vi "ConfigPhases.vi"(8 "error in (no error)":errorcluster, 11 "NhRegenGridSim in":refnum<class "NhRegenGridSim.lvclass">) -> (0 "error out":errorcluster, 3 "NhRegenGridSim out":refnum<class "NhRegenGridSim.lvclass">)   [LabVIEW 2018, in "AcPwrPlugins.lvlib" / "NhRegenGridSim.lvclass"]
doc: "This VI sets the selected logical instrument to apply changes at the set phase angle when operating with synchronization enabled using Configure Synchronization.vi.\n\nThis command ONLY applies to an instrument in AC mode."
uses:
  NhRegenGridSim.lvclass
  <instrlib>/NH Research 9400 Series/NH Research 9400 Series.lvlib
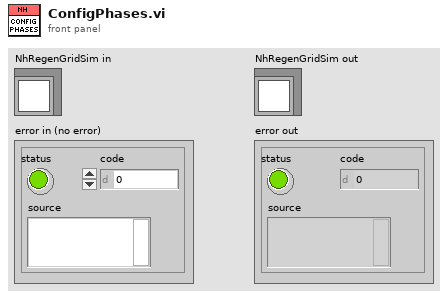
[diagram p1: front panel]
types:
  T1 = typedef "AcPwrPlugins.lvlib/NhRegenGridSim.lvclass/Load.ctl" = cluster{"SlewRates":cluster{"Islew":dbl, "Vslew":dbl, "Pslew":dbl, "FreqSlew":dbl, "AngleABSlew":dbl, "AngleACSlew":dbl}, "Phases":cluster{"Pout":dbl, "Iout":dbl, "PhaseAngle":dbl, "Vout":dbl, "Phase Name":string}[], "Measurement":cluster{"ApertureLength":dbl, "NumberOfSamples":u32}, "Ranges":cluster{"Irange":dbl, "Vrange":dbl}, "Mode":enum8{"One 3-Phase AC", "One AC", "One DC", "Three AC", "Three DC", "One 2-Phase AC and One AC", "One 2-Phase AC and One DC", "Two AC", "One AC and One DC", "Two AC and One DC", "One AC and Two DC", "One DC and One AC", "Two DC"}, "PowerMax":u16, "TransformerRatio":dbl, "Waveshape":dbl[], "Handle":string, "FreqOut":dbl, "Connected":bool, "Safety Limits":cluster{"Minimum Voltage (V)":dbl, "Minimum Voltage Time (s)":dbl, "Maximum Voltage (V)":dbl, "Maximum Voltage Time (s)":dbl, "Maximum Source Amps (A)":dbl, "Maximum Source Amps Time (s)":dbl, "Maximum Sink Amps (A)":dbl, "Maximum Sink Amps Time (s)":dbl, "Maximum Source Power (W)":dbl, "Maximum Source Power Time (s)":dbl, "Maximum Sink Power (W)":dbl, "Maximum Sink Power Time (s)":dbl, "Peak Voltage (V)":dbl, "Peak Voltage Enable":bool, "Peak Amps (A)":dbl, "Peak Amps Enable":bool}}
  T2 = enum8{"One 3-Phase AC", "One AC", "One DC", "Three AC", "Three DC", "One 2-Phase AC and One AC", "One 2-Phase AC and One DC", "Two AC", "One AC and One DC", "Two AC and One DC", "One AC and Two DC", "One DC and One AC", "Two DC"}
  T3 = cluster{"Pout":dbl, "Iout":dbl, "PhaseAngle":dbl, "Vout":dbl, "Phase Name":string}[]
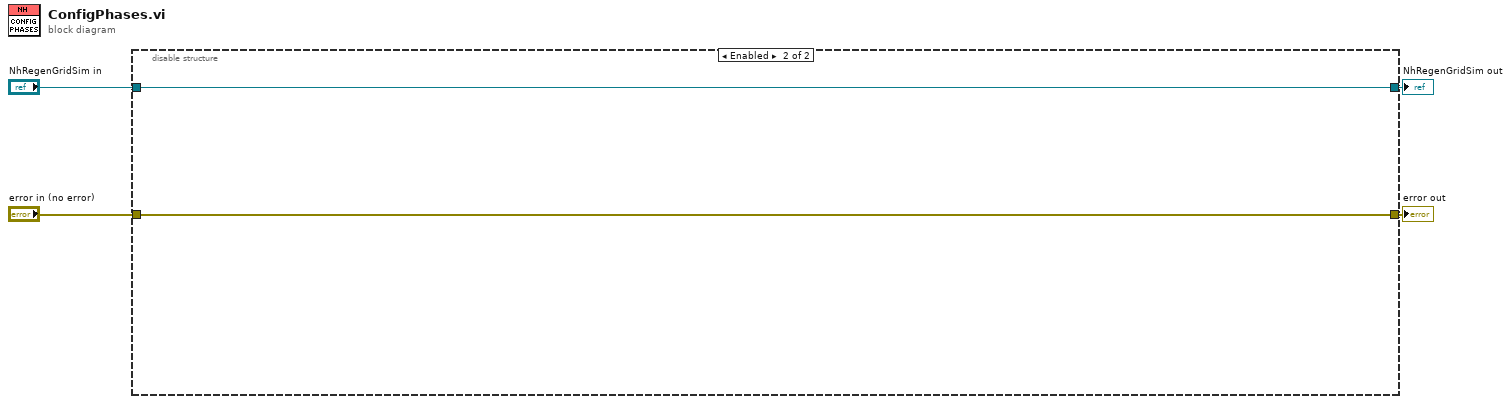
[diagram p0: block diagram]
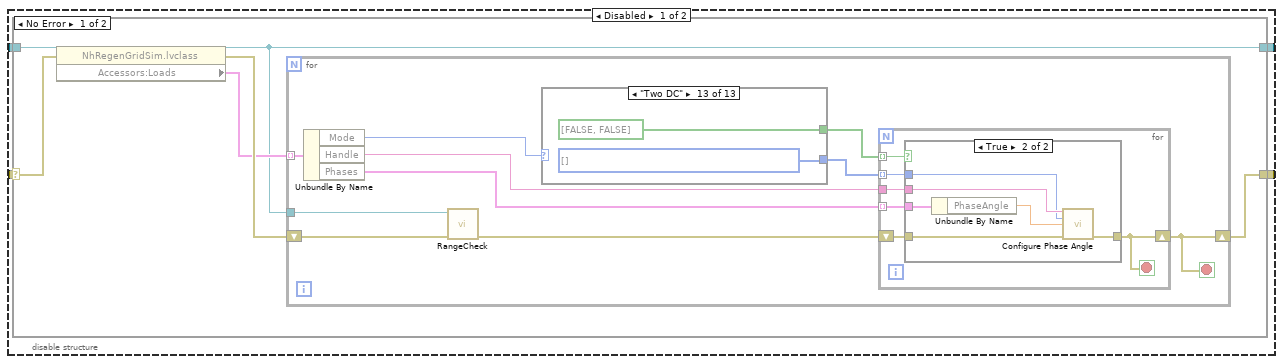
[diagram p2: hidden frame]
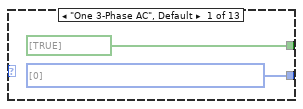
[diagram p3: hidden frame]
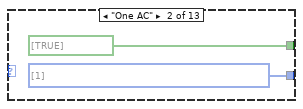
[diagram p4: hidden frame]
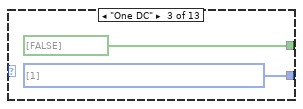
[diagram p5: hidden frame]
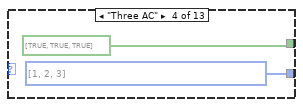
[diagram p6: hidden frame]
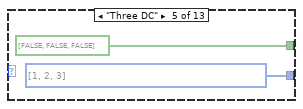
[diagram p7: hidden frame]
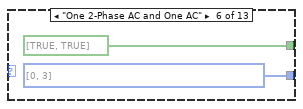
[diagram p8: hidden frame]
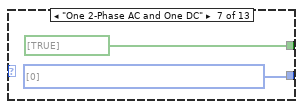
[diagram p9: hidden frame]
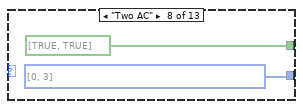
[diagram p10: hidden frame]
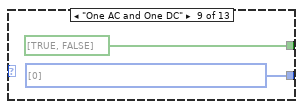
[diagram p11: hidden frame]
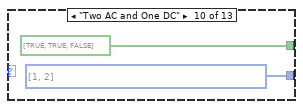
[diagram p12: hidden frame]
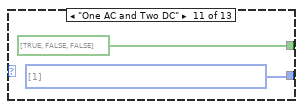
[diagram p13: hidden frame]
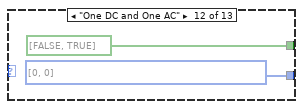
[diagram p14: hidden frame]
diagram:
  n1 = disable-structure shown="Enabled" {
    disable-tunnel: [w8 w66] -> w4
    disable-tunnel: [w7 w67] -> w3
    disable-tunnel: "error in (no error)" -> [w6 w66]
    disable-tunnel: "NhRegenGridSim in" -> [w5 w67]
    frame Disabled {
      n2 = case shown="No Error" w6 {
        selector: w6 -> [w13 w64]
        tunnel: [w11 w64] -> w8
        tunnel: [w9 w65] -> w7
        tunnel: w5 -> [w14 w65]
        frame No Error {
          n3 = property class="NhRegenGridSim.lvclass"(reference=w14, error in=w13) -> (reference out=w9:refnum<class "NhRegenGridSim.lvclass">, error out=w12:errorcluster, "Accessors:Loads"=w10:T1[])
          n4 = for {
            shift-right: [w18] -> w11
            shift-left: w12 -> [w21]
            tunnel: w10 -> [w23] mode=indexing
            tunnel: w9 -> [w19]
            stop <- w18 stop-if-true
            n5 = Unbundle By Name(w23) -> ("Mode"=w17:T2, "Handle"=w22:string, "Phases"=w24:T3)
            n6 = call-dynamic "RangeCheck.vi"("NhRegenGridSim in"=w19, "error in (no error)"=w21) -> ("error out"=w20:errorcluster)  [unwired: 7 in, 1 out]
            n7 = case shown="\"Two DC\"" w17 {
              tunnel: [w25 w28 w29 w32 w33 w35 w37 w39 w41 w43 w46 w48 w49] -> w15
              tunnel: [bool[] [TRUE] bool[] [TRUE] bool[] [FALSE] bool[] [TRUE, TRUE, TRUE] bool[] [FALSE, FALSE, FALSE] bool[] [TRUE, TRUE] bool[] [TRUE] bool[] [TRUE, TRUE] bool[] [TRUE, FALSE] bool[] [TRUE, TRUE, FALSE] bool[] [TRUE, FALSE, FALSE] bool[] [FALSE, TRUE] bool[] [FALSE, FALSE]] -> w16
              frame "One 3-Phase AC", Default {
                w25 = i32[] [0] items=["All", "A Phase", "B Phase", "C Phase"]
              }
              frame "One AC" {
                w28 = i32[] [1] items=["All", "A Phase", "B Phase", "C Phase"]
              }
              frame "One DC" {
                w29 = i32[] [1] items=["All", "A Phase", "B Phase", "C Phase"]
              }
              frame "Three AC" {
                w32 = i32[] [1, 2, 3] items=["All", "A Phase", "B Phase", "C Phase"]
              }
              frame "Three DC" {
                w33 = i32[] [1, 2, 3] items=["All", "A Phase", "B Phase", "C Phase"]
              }
              frame "One 2-Phase AC and One AC" {
                w35 = i32[] [0, 3] items=["All", "A Phase", "B Phase", "C Phase"]
              }
              frame "One 2-Phase AC and One DC" {
                w37 = i32[] [0] items=["All", "A Phase", "B Phase", "C Phase"]
              }
              frame "Two AC" {
                w39 = i32[] [0, 3] items=["All", "A Phase", "B Phase", "C Phase"]
              }
              frame "One AC and One DC" {
                w41 = i32[] [0] items=["All", "A Phase", "B Phase", "C Phase"]
              }
              frame "Two AC and One DC" {
                w43 = i32[] [1, 2] items=["All", "A Phase", "B Phase", "C Phase"]
              }
              frame "One AC and Two DC" {
                w46 = i32[] [1] items=["All", "A Phase", "B Phase", "C Phase"]
              }
              frame "One DC and One AC" {
                w48 = i32[] [0, 0] items=["All", "A Phase", "B Phase", "C Phase"]
              }
              frame "Two DC" {
                w49 = i32[] [] items=["All", "A Phase", "B Phase", "C Phase"]
              }
            }
            n8 = for {
              tunnel: w24 -> [w55] mode=indexing
              tunnel: w22 -> [w54]
              shift-right: [w53] -> w18
              shift-left: w20 -> [w56]
              tunnel: w16 -> [w52] mode=indexing
              tunnel: w15 -> [w51] mode=indexing
              stop <- w53 stop-if-true
              n9 = case shown="True" w52 {
                tunnel: w56 -> [w57 w63]
                tunnel: w55 -> [_ w62]
                tunnel: w54 -> [_ w60]
                tunnel: [w57 w59] -> w53
                tunnel: w51 -> [_ w58]
                frame False {
                }
                frame True {
                  n10 = Unbundle By Name(w62) -> ("PhaseAngle"=w61:dbl)
                  n11 = call <instrlib>:"Configure Phase Angle.vi"("VISA resource name"=w60, "Phase (0: All)"=w58, "Phase Angle (0 Degrees)"=w61, "error in (no error)"=w63) -> ("error out"=w59:errorcluster)  [unwired: 10 in, 1 out]
                }
              }
            }
          }
        }
        frame Error {
        }
      }
    }
    frame Enabled {
    }
  }
  "error out" <- w4
  "NhRegenGridSim out" <- w3
